vi "Main.vi"(8 "Error In":errorcluster) -> (0 "Error Out":errorcluster)   [LabVIEW 2017, in "Example Module.lvlib"]
uses:
  Example Module.lvlib
  Controls/Params.ctl
  Monochromator/Controls/Grating.ctl
  Monochromator/Controls/VISA parameters.ctl
  System Control/Main controller.lvlib
  Events/Events.lvlib
  Serial comms/Serial comms.lvlib
  Monochromator/Monochromator.lvlib
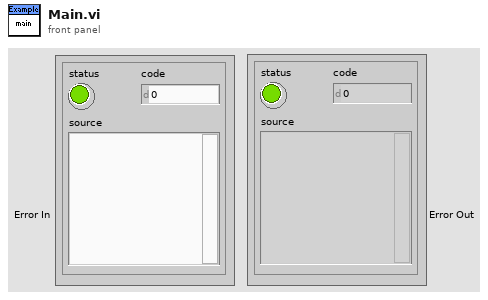
[diagram p1: front panel]
types:
  T1 = typedef "Example Module.lvlib/Params.ctl" = cluster{"Type":enum32{"Oriel", "PTI"}, "Wavelength (nm)":dbl, "Wavelength (nm)":string, "Grating, gr/mm":u16, "Grating mode":T2, "Spectrum mode":cluster{"Spectrum mode?":bool, "Start wavelength (nm)":dbl, "End wavelength (nm)":dbl, "Wavelength step (nm)":dbl, "Wavelength array":dbl[], "array index":u32}, "VISA":cluster{"delay before read (ms)":u32, "Mono 1":T3, "Mono 2":T3}}
  T2 = typedef "Monochromator.lvlib/Grating.ctl" = enum32{"Unknown", "Visible", "IR"}
  T3 = typedef "Serial comms.lvlib/VISA parameters.ctl" = cluster{"Timeout (ms)":u32, "Resource Name":refnum<visa-resource-name>, "Baud Rate":u32, "Data Bits":u16, "Parity":u16, "Stop Bits":u16, "Flow Control":u16}
  T4 = typedef "Events.lvlib/Refs [cluster].ctl" = cluster{"Exit":refnum<user-event>, "Controller":refnum<user-event>, "System Error":refnum<user-event>, "UI":refnum<user-event>, "Example Module":refnum<user-event>, "Shutter":refnum<user-event>, "Monochromator":refnum<user-event>, "DAQ":refnum<user-event>, "Scope":refnum<user-event>, "Processing":refnum<user-event>, "File IO":refnum<user-event>, "Colour wheel":refnum<user-event>}
  T5 = typedef "Example Module.lvlib/Commands [enum].ctl" = enum16{"Start", "Stop", "Send config"}
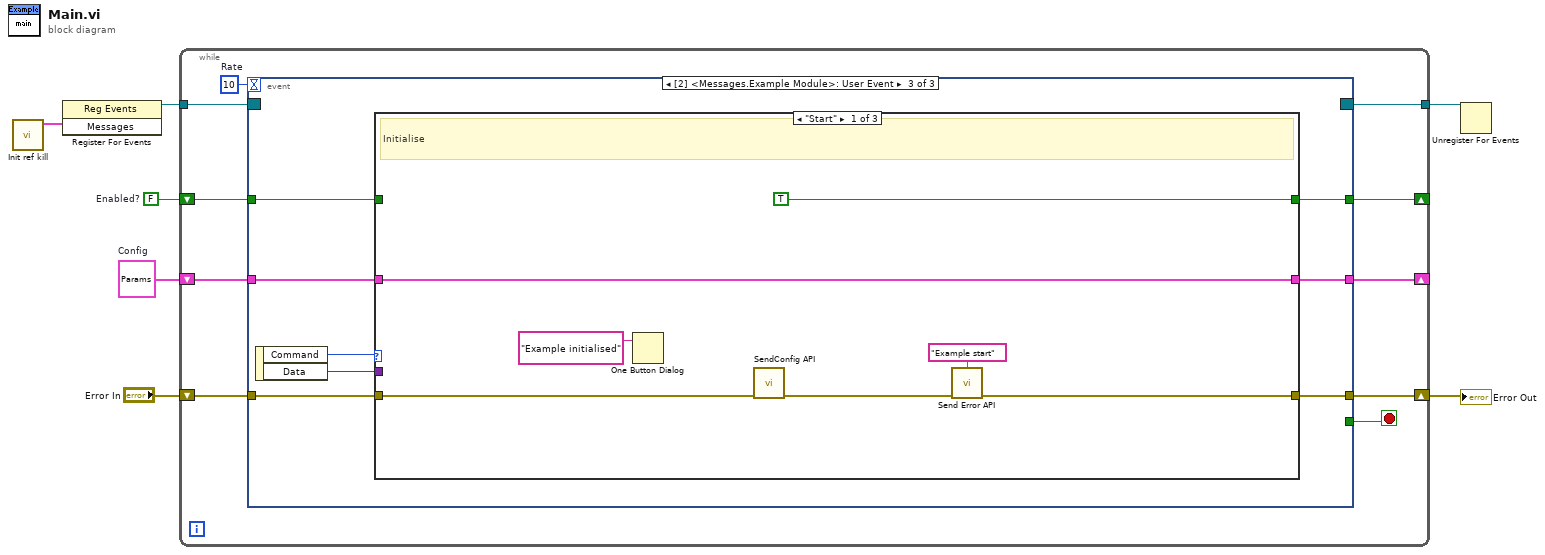
[diagram p0: block diagram]
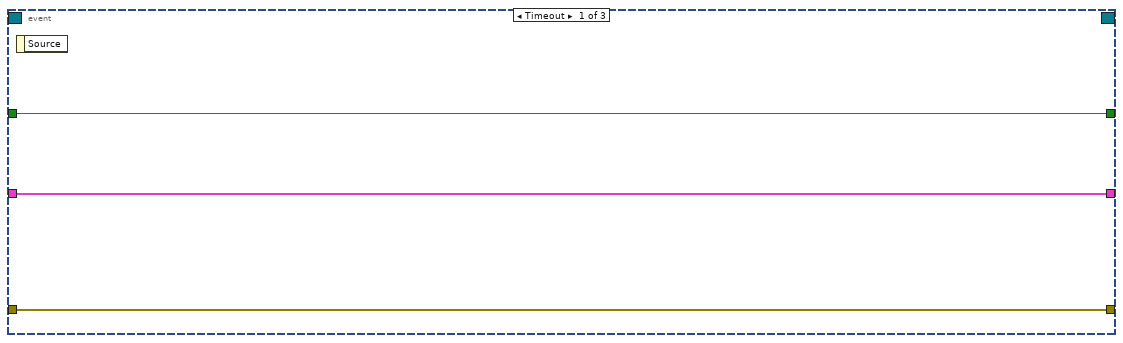
[diagram p2: hidden frame]
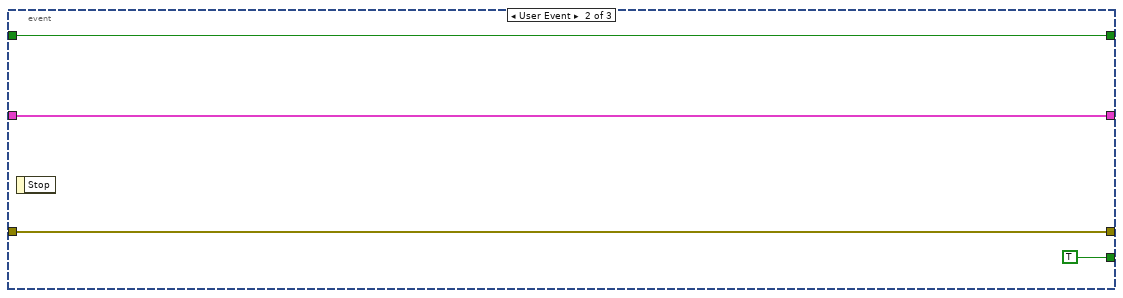
[diagram p3: hidden frame]
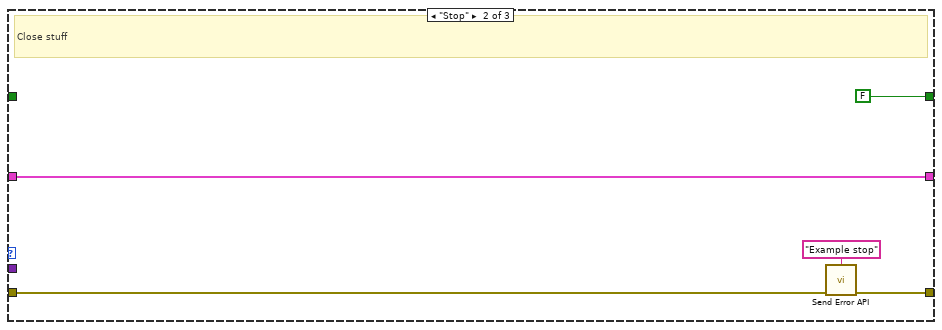
[diagram p4: hidden frame]
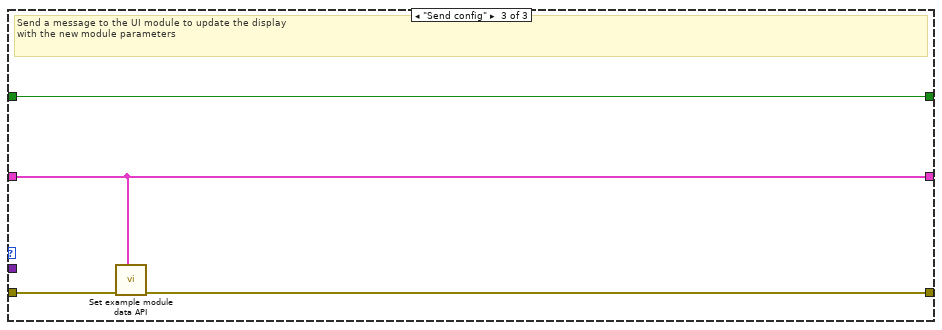
[diagram p5: hidden frame]
diagram:
  w1 = T1 {"Type"=enum."PTI", "Wavelength (nm)"=600.0, "Wavelength (nm)"="600 nm", "Grating, gr/mm"=2, "Grating mode"=enum."Unknown", "Spectrum mode"={"Spectrum mode?"=FALSE, "Start wavelength (nm)"=0.0, "End wavelength (nm)"=0.0, "Wavelength step (nm)"=0.0, "Wavelength array"=[], "array index"=0}, "VISA"={"delay before read (ms)"=50, "Mono 1"={"Timeout (ms)"=1000, "Resource Name"="COM1", "Baud Rate"=9600, "Data Bits"=8, "Parity"=0, "Stop Bits"=10, "Flow Control"=0}, "Mono 2"={"Timeout (ms)"=1000, "Resource Name"="COM1", "Baud Rate"=9600, "Data Bits"=8, "Parity"=0, "Stop Bits"=10, "Flow Control"=0}}}  # Config
  w5 = FALSE  # Enabled?
  n1 = call "Init ref kill.vi"() -> ("Messages"=w7:T4)  [unwired: 10 in, 1 out]
  n2 = register-events(w7) -> (reference out=w6:refnum<event-registration>)  [unwired: 2 in, 1 out]
  n3 = while {
    tunnel: w6 -> [w17]
    shift-right: [w13] -> _
    shift-left: w5 -> [w12]
    tunnel: [w14] -> w4
    shift-right: [w8] -> w2
    shift-left: "Error In" -> [w11]
    shift-right: [w9] -> _
    shift-left: w1 -> [w10]
    stop <- w15 stop-if-true
    w16 = 10  # Rate
    n4 = event shown="[2] <Messages.Example Module>: User Event" {
      selector: w17 -> [_ _ _]
      dyn-events: [_ _ _] -> w14
      timeout: w16 -> [_ _ _]
      tunnel: [_ TRUE _] -> w15
      tunnel: [w18 w21 w31] -> w13
      tunnel: w12 -> [w18 w21 w30]
      tunnel: w11 -> [w19 w22 w28]
      tunnel: [w19 w22 w27] -> w8
      tunnel: w10 -> [w20 w23 w26]
      tunnel: [w20 w23 w25] -> w9
      event Timeout {
        n5 = event-data() -> ()  [unwired: 1 in, 1 out]
      }
      event User Event {
        n6 = event-data() -> ()  [unwired: 1 in, 1 out]
      }
      event User Event {
        n7 = event-data() -> ("Command"=w32:T5, "Data"=w29:variant)  [unwired: 1 in]
        n8 = case shown="\"Start\"" w32 {
          tunnel: [TRUE FALSE w45] -> w31
          tunnel: w30 -> [_ _ w45]
          tunnel: w29 -> [_ _ _]
          tunnel: w28 -> [w33 w40 w48]
          tunnel: [w37 w42 w47] -> w27
          tunnel: w26 -> [w34 w43 w46]
          tunnel: [w34 w43 w46] -> w25
          frame "Start" {
            # "Initialise"
            n9 = One Button Dialog(message="Example initialised") -> ()  [unwired: 1 in, 1 out]
            n10 = call "SendConfig API.vi"("Error In"=w33) -> ("Error Out"=w38:errorcluster)  [unwired: 10 in]
            n11 = call "Send Error API.vi"("Error Cluster"=w38, "Error"="Example start") -> ("Error Out"=w37:errorcluster)  [unwired: 9 in]
          }
          frame "Stop" {
            # "Close stuff"
            n12 = call "Send Error API.vi"("Error Cluster"=w40, "Error"="Example stop") -> ("Error Out"=w42:errorcluster)  [unwired: 9 in]
          }
          frame "Send config" {
            # "Send a message to the UI module to update the display \nwith the new module parameters"
            n13 = call "Set example module data API.vi"("Config"=w46, "Error In"=w48) -> ("Error Out"=w47:errorcluster)  [unwired: 9 in]
          }
        }
      }
    }
  }
  "Error Out" <- w2
  n14 = Unregister For Events(event registration refnum=w4) -> ()  [unwired: 1 in, 1 out]
